vi "User@VIClose__Parameter.vi"(1 "ParamterIn":string) -> (0 "ParamterOut":string)   [LabVIEW 2020]
uses:
  MainFrame/Global.vi
panel:
  in  "VI":string(combo)
  in  "Confirm":bool
  # "User@VIClose $VI"
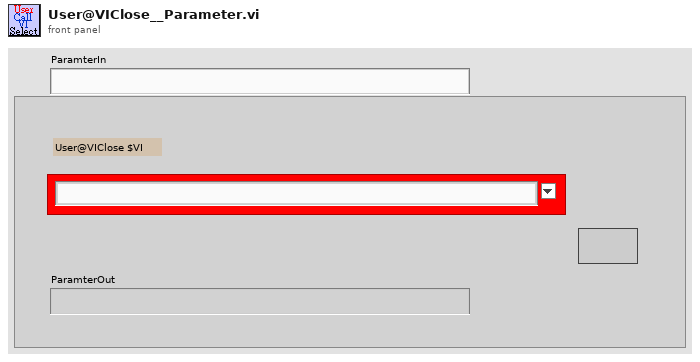
[diagram p1: front panel]
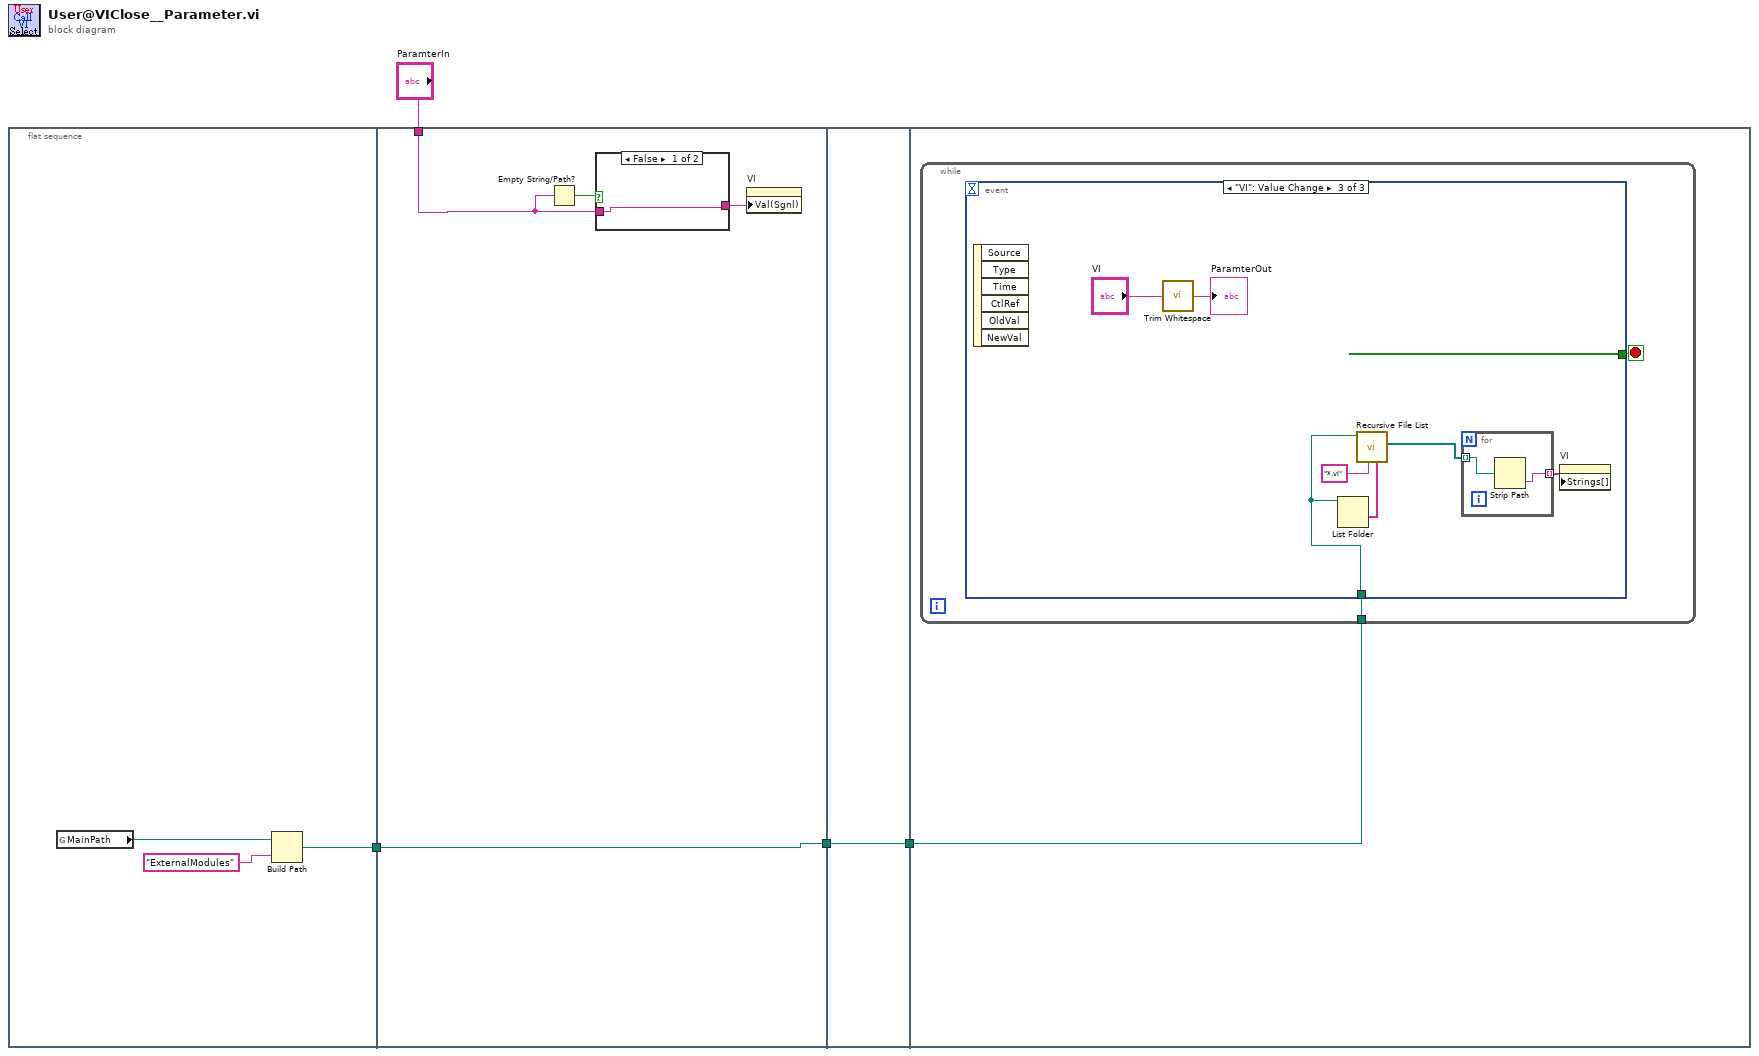
[diagram p0: block diagram]
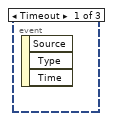
[diagram p3: hidden frame]
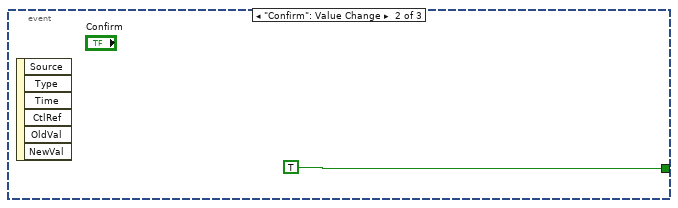
[diagram p4: hidden frame]
diagram:
  n1 = flat-sequence {
    tunnel: [w6] -> w1
    tunnel: "ParamterIn" -> [w8]
    tunnel: [w10] -> w2
    tunnel: w1 -> [w10]
    tunnel: [w14] -> w3
    tunnel: w2 -> [w14]
    tunnel: w3 -> [w15]
    frame #0 {
      n2 = global read "Global.vi" "MainPath"() -> (w5:path)
      n3 = Build Path(base path=w5, name or relative path="ExternalModules") -> (appended path=w6:path)
    }
    frame #1 {
      n4 = Empty String/Path?(string/path=w8) -> (empty?=w11:bool)
      n5 = case shown="False" w11 {
        tunnel: w8 -> [w12 w13]
        tunnel: [w12 w13] -> w9
        frame False {
        }
        frame True {
        }
      }
      n6 = property on="VI" class="CmbBox"("Val(Sgnl)"=w9) -> ()  [unwired: 2 in, 2 out]
    }
    frame #2 {
    }
    frame #3 {
      n7 = while {
        tunnel: w15 -> [w16]
        stop <- w17 stop-if-true
        n8 = event shown="[2] \"VI\": Value Change" {
          selector: _ -> [_ _ _]
          dyn-events: _ -> [_ _ _]
          timeout: _ -> [_ _ _]
          tunnel: [_ TRUE _] -> w17
          tunnel: w16 -> [_ _ w22]
          event Timeout {
            n9 = event-data() -> ()  [unwired: 1 in, 3 out]
          }
          event "Confirm": Value Change {
            n10 = event-data() -> ()  [unwired: 1 in, 6 out]
          }
          event "VI": Value Change {
            n11 = event-data() -> ()  [unwired: 1 in, 6 out]
            n12 = call <vilib>:"Trim Whitespace.vi"("string"="VI") -> ("trimmed string"=→"ParamterOut":string)  [unwired: 1 in]
            n13 = List Folder(path=w22) -> (folder names=w21:string[])  [unwired: 3 in, 3 out]
            n14 = call <vilib>:"Recursive File List.vi"("Folders to Exclude"=w21, "pattern"="*.vi", "Folder Path"=w22) -> ("All Files in Dir"=w25:path[])  [unwired: 4 in, 4 out]
            n15 = for {
              tunnel: w25 -> [w27] mode=indexing
              tunnel: [w26] -> w23 mode=indexing
              n16 = Strip Path(path=w27) -> (name=w26:string)  [unwired: 1 out]
            }
            n17 = property on="VI" class="CmbBox"("Strings[]"=w23) -> ()  [unwired: 2 in, 2 out]
          }
        }
      }
    }
  }
